vi "SyringePump.vi"() -> ()   [LabVIEW 2018]
doc: "Demonstrates interactive control on the pump. User can interactively control the operation on the pump such as infuse, pause, withdraw and stop. \nThis VI continously output the status and the delivered volume.\n\n<b>Note:</b>\n- The pump does not support remote syringe volume setting. User must set the syringe volume on the pump before running this example. The Target Volume must be less than or equal to the syringe volume. \n- Does not work with Serial Interface. Delays need to be added for Serial Interface."
uses:
  <instrlib>/Harvard Apparatus PHD Ultra Series/Harvard Apparatus PHD Ultra Series.lvlib
panel:
  out "Withdrawn volume units":string
  out "Infused volume units":string
  out "Infused Volume":dbl
  out "Withdrawn Volume":dbl
  out "Infuse Units":u16(ring)=1 items=["milliliters", "microliters", "nanoliters", "picoliters"]
  out "Withdraw Units":u16(ring)=1 items=["milliliters", "microliters", "nanoliters", "picoliters"]
  in  "# Syringes":i32=1
  in  "stop":bool
  in  "Syringe Diameter (20 mm)":dbl=44.0 min=1.0 max=99.0 format="%#.3f"
  in  "Tab Control":enum32{"Steady", "Ramp"}(tab)
  in  "Flow Rate (5)":dbl=5.0 format="%#.4f"
  in  "Flow Rate Units (1:ml/min)":u32(ring)=1 items=["milliliters per hour (ml/hr)", "milliliters per minute (ml/min)", "milliliters per second (ml/sec)", "microliters per hour (ul/hr)", "microliters per minute (ul/min)", "microliters per second (ul/sec)", "nanoliters per hour (nl/hr)", "nanoliters per minute (nl/min)", "nanoliters per second (nl/sec)", "picoliters per hour (pl/hr)", "picoliters per minute (pl/min)", "picoliters per second (pl/sec)"]
  in  "Pause":bool
  in  "Start":bool
  in  "Run Method (0:Infuse)":u16(ring)=1 items=["Infuse", "Withdraw"]
  in  "Initial Flow Rate (5.00)":dbl=5.0 format="%#.4f"
  in  "Pump Direction (0:Infuse)":u16(ring)=1 items=["Infuse", "Withdraw"]
  in  "Infuse Time":dbl=5.0 format="%#.4f"
  in  "Final Flow Rate (5.00)":dbl=50.0 format="%#.4f"
  in  "Flow Rate Units (1:ml/min) 2":u32(ring)=1 items=["milliliters per hour (ml/hr)", "milliliters per minute (ml/min)", "milliliters per second (ml/sec)", "microliters per hour (ul/hr)", "microliters per minute (ul/min)", "microliters per second (ul/sec)", "nanoliters per hour (nl/hr)", "nanoliters per minute (nl/min)", "nanoliters per second (nl/sec)", "picoliters per hour (pl/hr)", "picoliters per minute (pl/min)", "picoliters per second (pl/sec)"]
  in  "Start Ramp":bool
  in  "Baud Rate (115200)":u32(ring)=115200 items=["9600"=9600, "19200"=19200, "38400"=38400, "57600"=57600, "115200"=115200]
  out "Idle":bool
  out "Withdrawing":bool
  out "Infusing":bool
  in  "Stop":bool
  in  "VISA resource name":refnum<visa-resource-name>="COM25"
  # "NOTE: The flow rate is compensated for the number of syringes in the code"
  # "Status"
  # "Controls"
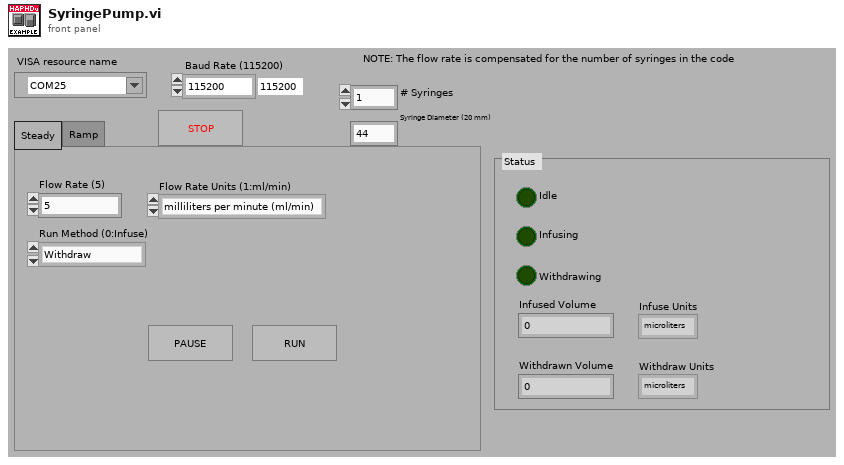
[diagram p1: front panel]
types:
  T1 = enum16{"open", "open or create", "create or replace", "create", "open (read-only)"}
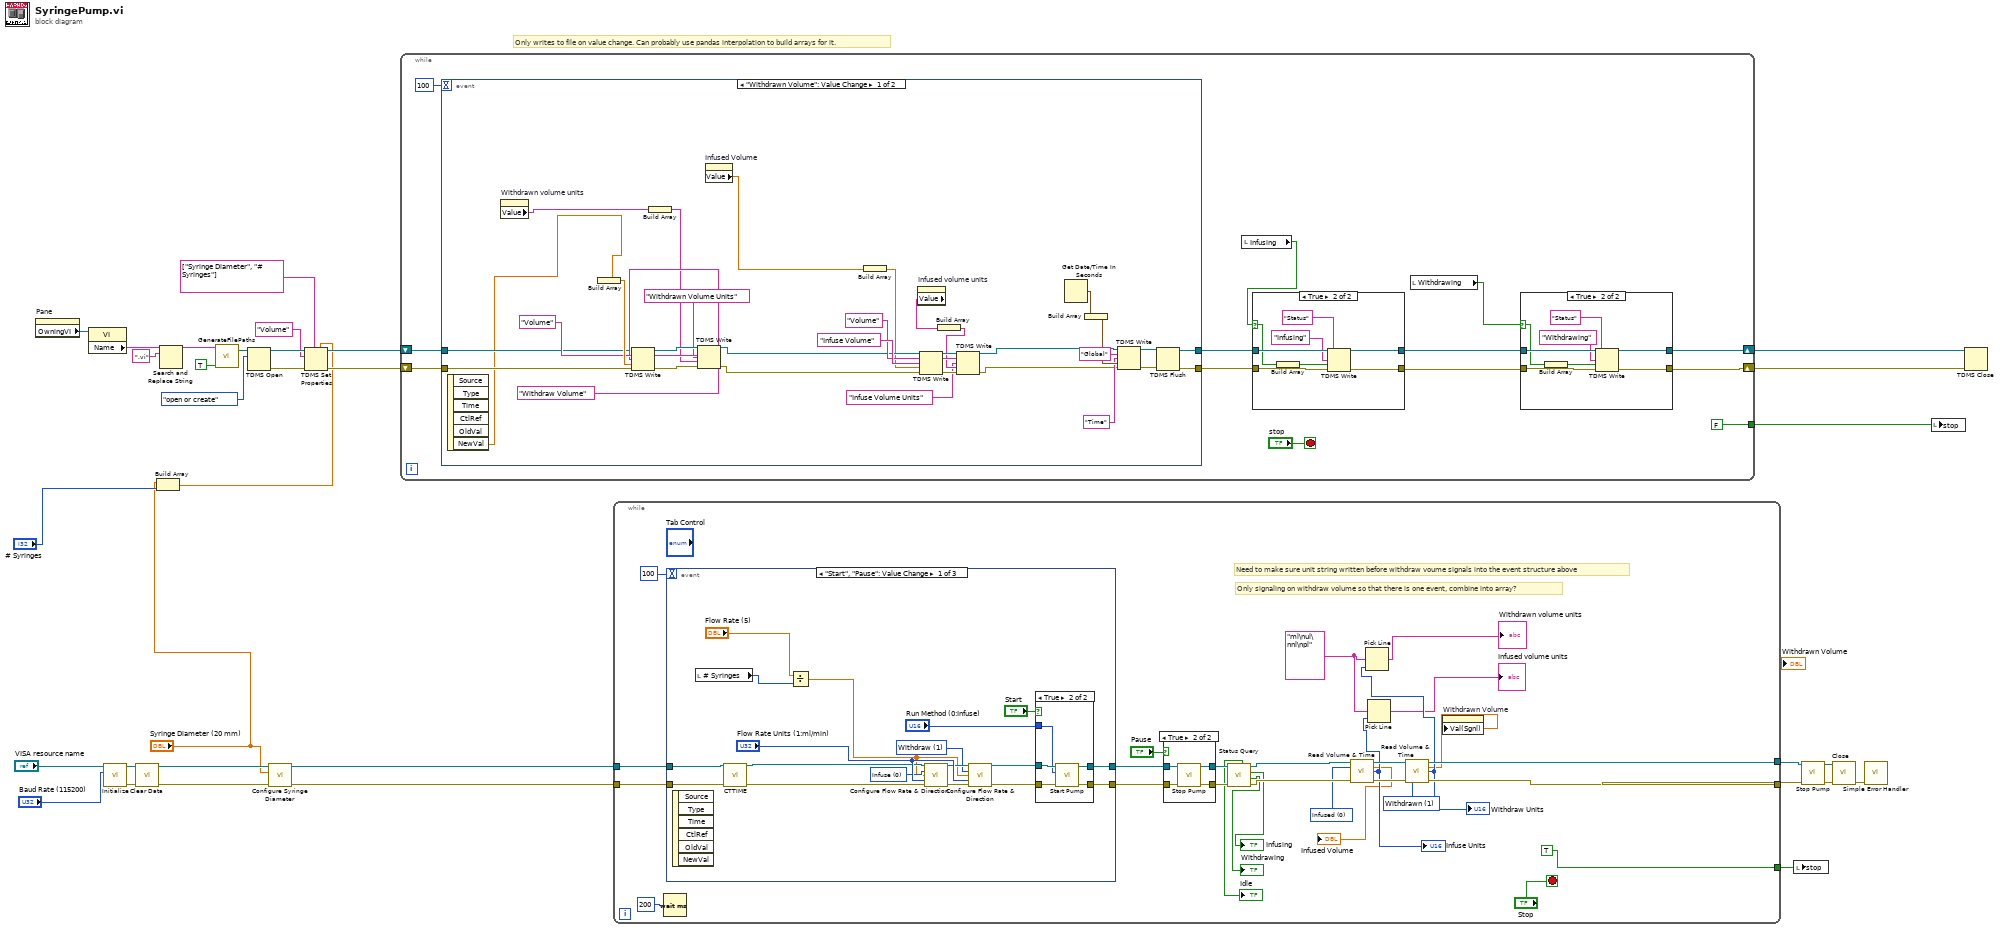
[diagram p0: block diagram]
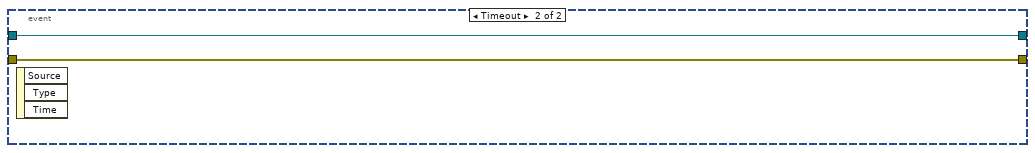
[diagram p4: hidden frame]
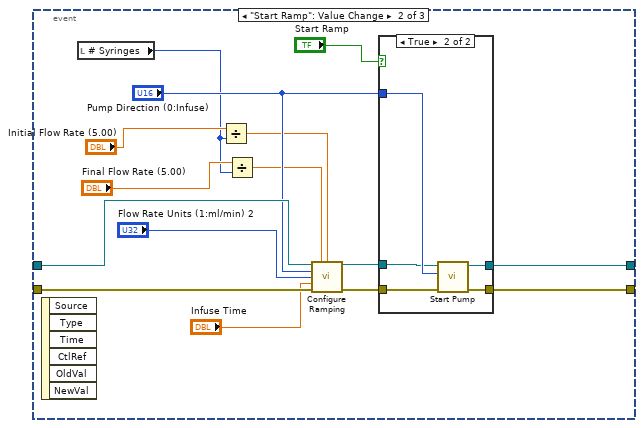
[diagram p7: hidden frame]
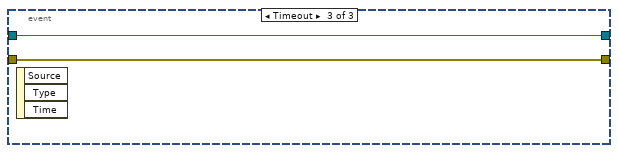
[diagram p9: hidden frame]
diagram:
  # "Only writes to file on value change. Can probably use pandas interpolation to build arrays for it."
  n1 = property on="Pane" class="Pane"() -> ("OwningVI"=w20:refnum<vi>)  [unwired: 2 in, 2 out]
  n2 = property class="VI"(reference=w20) -> ("Name"=w16:string)  [unwired: 1 in, 2 out]
  n3 = call <instrlib>:"Initialize.vi"("Baud Rate (115200)"="Baud Rate (115200)", "VISA resource name"="VISA resource name") -> ("error out"=w32:errorcluster, "VISA resource name out"=w31:refnum<visa-resource-name>)  [unwired: 8 in]
  n4 = call <instrlib>:"Clear Data.vi"("error in (no error)"=w32, "VISA resource name"=w31) -> ("error out"=w29:errorcluster, "VISA resource name out"=w30:refnum<visa-resource-name>)  [unwired: 8 in]
  n5 = Build Array("Syringe Diameter (20 mm)", "# Syringes") -> (w1:dbl[])
  n6 = Search and Replace String(input string=w16, search string=".vi") -> (result string=w18:string)  [unwired: 6 in, 3 out]
  n7 = call "GenerateFilePaths.vi"("Logfile? (F)"=TRUE ("Logfile?"), "Device Name"=w18) -> ("Path"=w15:path)  [unwired: 3 in]
  n8 = TDMS Open(10:T1."open or create" ("operation (0:open)"), 11:w15) -> (0:w9:errorcluster, 3:w8:refnum<k34>)  [unwired: 5 in]
  n9 = call <instrlib>:"Configure Syringe Diameter.vi"("error in (no error)"=w29, "Syringe Diameter (20 mm)"="Syringe Diameter (20 mm)", "VISA resource name"=w30) -> ("error out"=w21:errorcluster, "VISA resource name out"=w22:refnum<visa-resource-name>)  [unwired: 7 in]
  n10 = TDMS Set Properties(5:w1, 7:string[] ["Syringe Diameter", "# Syringes"] ("group name in (Untitled)"), 8:w9, 10:"Volume" ("group name in (Untitled)"), 11:w8) -> (0:w6:errorcluster, 3:w7:refnum<k34>)  [unwired: 1 in, 2 out]
  n11 = while {
    shift-right: [w36] -> w13
    shift-left: w7 -> [w46]
    shift-right: [w37] -> w12
    shift-left: w6 -> [w45]
    tunnel: [FALSE] -> w10
    stop <- "stop" stop-if-true
    n12 = event shown="[0] \"Withdrawn Volume\": Value Change" {
      selector: _ -> [_ _]
      dyn-events: _ -> [_ _]
      timeout: 100 -> [_ _]
      tunnel: w46 -> [w90 w102]
      tunnel: w45 -> [w89 w101]
      tunnel: [w88 w102] -> w41
      tunnel: [w87 w101] -> w40
      event "Withdrawn Volume": Value Change {
        n13 = event-data() -> ("NewVal"=w86:dbl)  [unwired: 1 in, 5 out]
        n14 = property on="Withdrawn volume units" class="Str"() -> ("Value"=w83:string)  [unwired: 2 in, 2 out]
        n15 = Build Array(w86) -> (w96:dbl[])
        n16 = TDMS Write(0:w90, 5:"Volume" ("group name in (Untitled)"), 7:"Withdraw Volume", 9:w96, 11:w89) -> (4:w94:refnum<k34>, 6:w85:string, 15:w95:errorcluster)  [unwired: 1 in, 1 out]
        n17 = Build Array(w83) -> (w82:string[])
        n18 = TDMS Write(0:w94, 5:w85, 7:"Withdrawn Volume Units", 9:w82, 11:w95) -> (4:w73:refnum<k34>, 15:w71:errorcluster)  [unwired: 1 in, 2 out]
        n19 = property on="Infused Volume" class="DigNum (strict)"() -> ("Value"=w68:dbl)  [unwired: 2 in, 2 out]
        n20 = Build Array(w68) -> (w67:dbl[])
        n21 = property on="Infused volume units" class="Str"() -> ("Value"=w77:string)  [unwired: 2 in, 2 out]
        n22 = TDMS Write(0:w73, 5:"Volume" ("group name in (Untitled)"), 7:"Infuse Volume", 9:w67, 11:w71) -> (4:w79:refnum<k34>, 6:w80:string, 15:w78:errorcluster)  [unwired: 1 in, 1 out]
        n23 = Build Array(w77) -> (w76:string[])
        n24 = TDMS Write(0:w79, 5:w80, 7:"Infuse Volume Units" ("String"), 9:w76, 11:w78) -> (4:w72:refnum<k34>, 15:w70:errorcluster)  [unwired: 1 in, 2 out]
        n25 = Get Date/Time In Seconds() -> (seconds since 1Jan1904=w99:timestamp)
        n26 = Build Array(w99) -> (w100:timestamp[])
        n27 = TDMS Write(0:w72, 5:"Global" ("group name in (Untitled)"), 7:"Time", 9:w100, 11:w70) -> (4:w97:refnum<k34>, 15:w98:errorcluster)  [unwired: 1 in, 2 out]
        n28 = TDMS Flush(4:w98, 7:w97) -> (0:w87:errorcluster, 3:w88:refnum<k34>)
      }
      event Timeout {
        n29 = event-data() -> ()  [unwired: 1 in, 3 out]
      }
    }
    n30 = local read "Infusing"() -> (w39:bool)
    n31 = case shown="True" w39 {
      selector: w39 -> [_ w61]
      tunnel: w41 -> [w58 w66]
      tunnel: w40 -> [w57 w65]
      tunnel: [w57 w64] -> w38
      tunnel: [w58 w63] -> w35
      frame False {
      }
      frame True {
        n32 = Build Array(w61) -> (w59:bool[])
        n33 = TDMS Write(0:w66, 5:"Status" ("group name in (Untitled)"), 7:"Infusing", 9:w59, 11:w65) -> (4:w63:refnum<k34>, 15:w64:errorcluster)  [unwired: 1 in, 2 out]
      }
    }
    n34 = local read "Withdrawing"() -> (w34:bool)
    n35 = case shown="True" w34 {
      selector: w34 -> [_ w51]
      tunnel: w35 -> [w48 w56]
      tunnel: w38 -> [w47 w55]
      tunnel: [w47 w54] -> w37
      tunnel: [w48 w53] -> w36
      frame False {
      }
      frame True {
        n36 = Build Array(w51) -> (w49:bool[])
        n37 = TDMS Write(0:w56, 5:"Status" ("group name in (Untitled)"), 7:"Withdrawing", 9:w49, 11:w55) -> (4:w53:refnum<k34>, 15:w54:errorcluster)  [unwired: 1 in, 2 out]
      }
    }
  }
  n38 = while {
    tunnel: w22 -> [w131]
    tunnel: [w120] -> w25
    tunnel: [w119] -> w24
    tunnel: w21 -> [w128]
    tunnel: [TRUE] -> w11
    stop <- "Stop" stop-if-true
    w107 = "ml\nul\nnl\npl" ("multi-line string")
    w110 = u16 0 items=["Infused", "Withdrawn"] ("Pump Method (0:Infused)")
    w111 = u16 1 items=["Infused", "Withdrawn"] ("Pump Method (0:Infused)")
    # "Only signaling on withdraw volume so that there is one event, combine into array?"
    # "Need to make sure unit string written before withdraw voume signals into the event structure above"
    n39 = Wait (ms)(milliseconds to wait=u32 200) -> ()  [unwired: 1 out]
    n40 = event shown="[0] \"Start\", \"Pause\": Value Change" {
      selector: _ -> [_ _ _]
      dyn-events: _ -> [_ _ _]
      timeout: 100 -> [_ _ _]
      tunnel: w128 -> [w142 w173 w185]
      tunnel: w131 -> [w144 w174 w186]
      tunnel: [w154 w176 w186] -> w127
      tunnel: [w153 w175 w185] -> w126
      event "Start", "Pause": Value Change {
        w147 = u16 0 items=["Infuse", "Withdraw"] ("Pump Method (0:Infuse)")
        w148 = u16 1 items=["Infuse", "Withdraw"] ("Pump Method (0:Infuse)")
        n41 = event-data() -> ()  [unwired: 1 in, 6 out]
        n42 = local read "# Syringes"() -> (w139:i32)
        n43 = call <instrlib>:"CTTIME.vi"("VISA resource name"=w144, "error in (no error)"=w142) -> ("VISA resource name out"=w143:refnum<visa-resource-name>, "error out"=w141:errorcluster)  [unwired: 12 in]
        n44 = Divide(x="Flow Rate (5)", y=w139) -> (x/y=w138:dbl)
        n45 = call <instrlib>:"Configure Flow Rate & Direction.vi"("VISA resource name"=w143, "Pump Direction (0:Infuse)"=w147, "Flow Rate (5.00)"=w138, "Flow Rate Units (1:ml/min)"="Flow Rate Units (1:ml/min)", "error in (no error)"=w141) -> ("VISA resource name out"=w149:refnum<visa-resource-name>, "error out"=w151:errorcluster)  [unwired: 9 in]
        n46 = call <instrlib>:"Configure Flow Rate & Direction.vi"("VISA resource name"=w149, "Pump Direction (0:Infuse)"=w148, "Flow Rate (5.00)"=w138, "Flow Rate Units (1:ml/min)"="Flow Rate Units (1:ml/min)", "error in (no error)"=w151) -> ("VISA resource name out"=w146:refnum<visa-resource-name>, "error out"=w145:errorcluster)  [unwired: 9 in]
        n47 = case shown="True" "Start" {
          tunnel: w146 -> [w157 w162]
          tunnel: w145 -> [w156 w161]
          tunnel: [w157 w160] -> w154
          tunnel: [w156 w159] -> w153
          tunnel: "Run Method (0:Infuse)" -> [_ w158]
          frame False {
          }
          frame True {
            n48 = call <instrlib>:"Start Pump.vi"("error in (no error)"=w161, "Run Direction (0:Infuse)"=w158, "VISA resource name"=w162) -> ("error out"=w159:errorcluster, "VISA resource name out"=w160:refnum<visa-resource-name>)  [unwired: 7 in]
          }
        }
      }
      event "Start Ramp": Value Change {
        n49 = event-data() -> ()  [unwired: 1 in, 6 out]
        n50 = local read "# Syringes"() -> (w163:i32)
        n51 = Divide(x="Initial Flow Rate (5.00)", y=w163) -> (x/y=w164:dbl)
        n52 = Divide(x="Final Flow Rate (5.00)", y=w163) -> (x/y=w165:dbl)
        n53 = call <instrlib>:"Configure Ramping.vi"("VISA resource name"=w174, "End Rate (10.00)"=w165, "Start Rate (5.00)"=w164, "Pump Method (0:Infuse)"="Pump Direction (0:Infuse)", "Flow Rate Units (1:ml/min)"="Flow Rate Units (1:ml/min) 2", "Ramp Time (10 seconds)"="Infuse Time", "error in (no error)"=w173) -> ("VISA resource name out"=w171:refnum<visa-resource-name>, "error out"=w172:errorcluster)  [unwired: 7 in]
        n54 = case shown="True" "Start Ramp" {
          tunnel: "Pump Direction (0:Infuse)" -> [_ w184]
          tunnel: w171 -> [w179 w183]
          tunnel: w172 -> [w178 w182]
          tunnel: [w179 w181] -> w176
          tunnel: [w178 w180] -> w175
          frame False {
          }
          frame True {
            n55 = call <instrlib>:"Start Pump.vi"("error in (no error)"=w182, "Run Direction (0:Infuse)"=w184, "VISA resource name"=w183) -> ("error out"=w180:errorcluster, "VISA resource name out"=w181:refnum<visa-resource-name>)  [unwired: 7 in]
          }
        }
      }
      event Timeout {
        n56 = event-data() -> ()  [unwired: 1 in, 3 out]
      }
    }
    n57 = case shown="True" "Pause" {
      tunnel: w127 -> [w133 w137]
      tunnel: w126 -> [w132 w136]
      tunnel: [w133 w135] -> w124
      tunnel: [w132 w134] -> w125
      frame False {
      }
      frame True {
        n58 = call <instrlib>:"Stop Pump.vi"("error in (no error)"=w136, "VISA resource name"=w137) -> ("error out"=w134:errorcluster, "VISA resource name out"=w135:refnum<visa-resource-name>)  [unwired: 8 in]
      }
    }
    n59 = call <instrlib>:"Status Query.vi"("error in (no error)"=w125, "VISA resource name"=w124) -> ("error out"=w118:errorcluster, "Withdrawing"=→"Withdrawing":bool, "Infusing"=→"Infusing":bool, "VISA resource name out"=w117:refnum<visa-resource-name>, "Idle"=→"Idle":bool)  [unwired: 4 in, 1 out]
    n60 = call <instrlib>:"Read Volume & Time .vi"("VISA resource name"=w117, "Pump Direction (0:Infused)"=w110, "error in (no error)"=w118) -> ("VISA resource name out"=w112:refnum<visa-resource-name>, "Volume"=→"Infused Volume":dbl, "Volume Units"=w109:u16, "error out"=w113:errorcluster)  [unwired: 7 in, 2 out]
    "Infuse Units" <- w109
    n61 = Pick Line(multi-line string=w107, line index=w109) -> (output string=→"Infused volume units":string)  [unwired: 1 in]
    n62 = call <instrlib>:"Read Volume & Time .vi"("VISA resource name"=w112, "Pump Direction (0:Infused)"=w111, "error in (no error)"=w113) -> ("VISA resource name out"=w120:refnum<visa-resource-name>, "Volume"=w105:dbl, "Volume Units"=w108:u16, "error out"=w119:errorcluster)  [unwired: 7 in, 2 out]
    "Withdraw Units" <- w108
    n63 = Pick Line(multi-line string=w107, line index=w108) -> (output string=→"Withdrawn volume units":string)  [unwired: 1 in]
    n64 = property on="Withdrawn Volume" class="DigNum (strict)"("Val(Sgnl)"=w105) -> ()  [unwired: 2 in, 2 out]
  }
  n65 = local write "stop"(w11) -> ()
  n66 = call <instrlib>:"Stop Pump.vi"("error in (no error)"=w24, "VISA resource name"=w25) -> ("error out"=w28:errorcluster, "VISA resource name out"=w27:refnum<visa-resource-name>)  [unwired: 8 in]
  n67 = call <instrlib>:"Close.vi"("error in (no error)"=w28, "VISA resource name"=w27) -> ("error out"=w26:errorcluster)  [unwired: 9 in]
  n68 = call <vilib>:"Simple Error Handler.vi"("error in (no error)"=w26) -> ()  [unwired: 4 in, 5 out]
  n69 = local write "stop"(w10) -> ()
  n70 = TDMS Close(8:w12, 11:w13) -> ()  [unwired: 2 out]
